vi "to_td_array.vi"(11 "TypeDescriptor in":refnum<class "TD.lvclass">) -> (3 "type string":i16[](array[numeric]))   [LabVIEW 2020, in "variant.lvlib" / "type.lvlib" / "TD.lvclass"]
uses:
  TD.lvclass
  C:/projects/OpenG-Variant-Data-Library/source/library/Bytes/Bytes.lvclass
  Bytes/Bytes.lvclass/Bytes.ctl
  Bytes/Bytes.lvclass
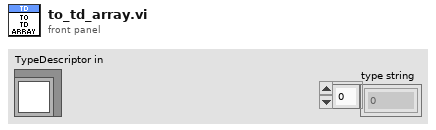
[diagram p1: front panel]
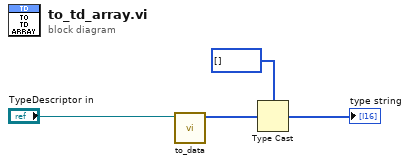
[diagram p0: block diagram]
diagram:
  n1 = call "to_data.vi"("Bytes in"="TypeDescriptor in") -> ("byte array"=w1:u8[])  [unwired: 10 in]
  n2 = Type Cast(type=i16[] [] ("type string"), x=w1) -> (*(type *) &x=→"type string":i16[])
